vi "Data_get_joe_3.vi"() -> ()   [LabVIEW 2011]
uses:
  <vilib>/Utility/error.llb/DialogType.ctl
  <vilib>/Analysis/2dsp.llb/Real FFT.vi
  <vilib>/Analysis/NI_AALPro.lvlib
panel:
  in  "Automatic Overwrite?":bool
  out "f cur. (GHz)":i32
  in  "TDS VISA Port":refnum<visa-resource-name>="GPIB0::1::INSTR"
  in  "Chirp up to (GHz)":dbl
  in  "PauseB":bool caption="Pause"
  in  "Substr":bool
  out "tdsavges#":i32 caption="tds averaged:"
  in  "Auto":bool caption="Autosave"
  in  "FFT every#":u32=1 min=1 max=1000 step=1
  in  "#steps":u32=1 min=1 step=1
  in  "f step (GHz)":dbl=0.0003 min=0.00025 max=67.0 step=1e-06 format="%#.12f"
  in  "time/point":T1(ring)
  in  "time/div":T2(ring)
  out "Current sweep":u32=1 min=1 max=1000 step=1
  in  "Ext":string="ccd"
  in  "Name":string="trace"
  in  "Folder":path
  in  "#Sweeps":u32=1 min=1 max=1000 step=1
  in  "Ampl. (dBm)":dbl min=-135.0 max=30.0 step=0.5 format="%#_8g"
  in  "f start (GHz)":dbl=0.0003 min=0.00025 max=67.0 step=1e-06 format="%#.12f"
  in  "Start":bool
  in  "Quit":bool
  in  "PSG1 VISA Port":refnum<visa-resource-name>="GPIB0::1::INSTR"
  out "read time (ms)":u32
  out "#points":u32
  out "Busy":bool
  in  "Chirp start (MHz)":ext=2.5
  in  "Filter up to (MHz)":ext=2.5
  in  "Amount of averagings":u32=10 min=1 step=1
  out "Data":dbl[](array[numeric])
  out "Frequency Domain Signal":cluster{ext[], dbl[]}(graph)
  out "FFT (Im)":dbl[](array[numeric])
  out "FFT (Re)":dbl[](array[numeric])
  out "Final array":ext[][](array[numeric])
  out "size(s)":i32
  out "Oscilloscope Data":dbl[](array[numeric])
  in  "Channel Number":u16=1
  out "Oscilloscope graph":dbl[](graph)
  in  "Stop":bool
  # "Oscilloscope TDS6124C"
  # "File Storage"
  # "PSG E8257D"
  # "Control"
  # "Spectrum data"
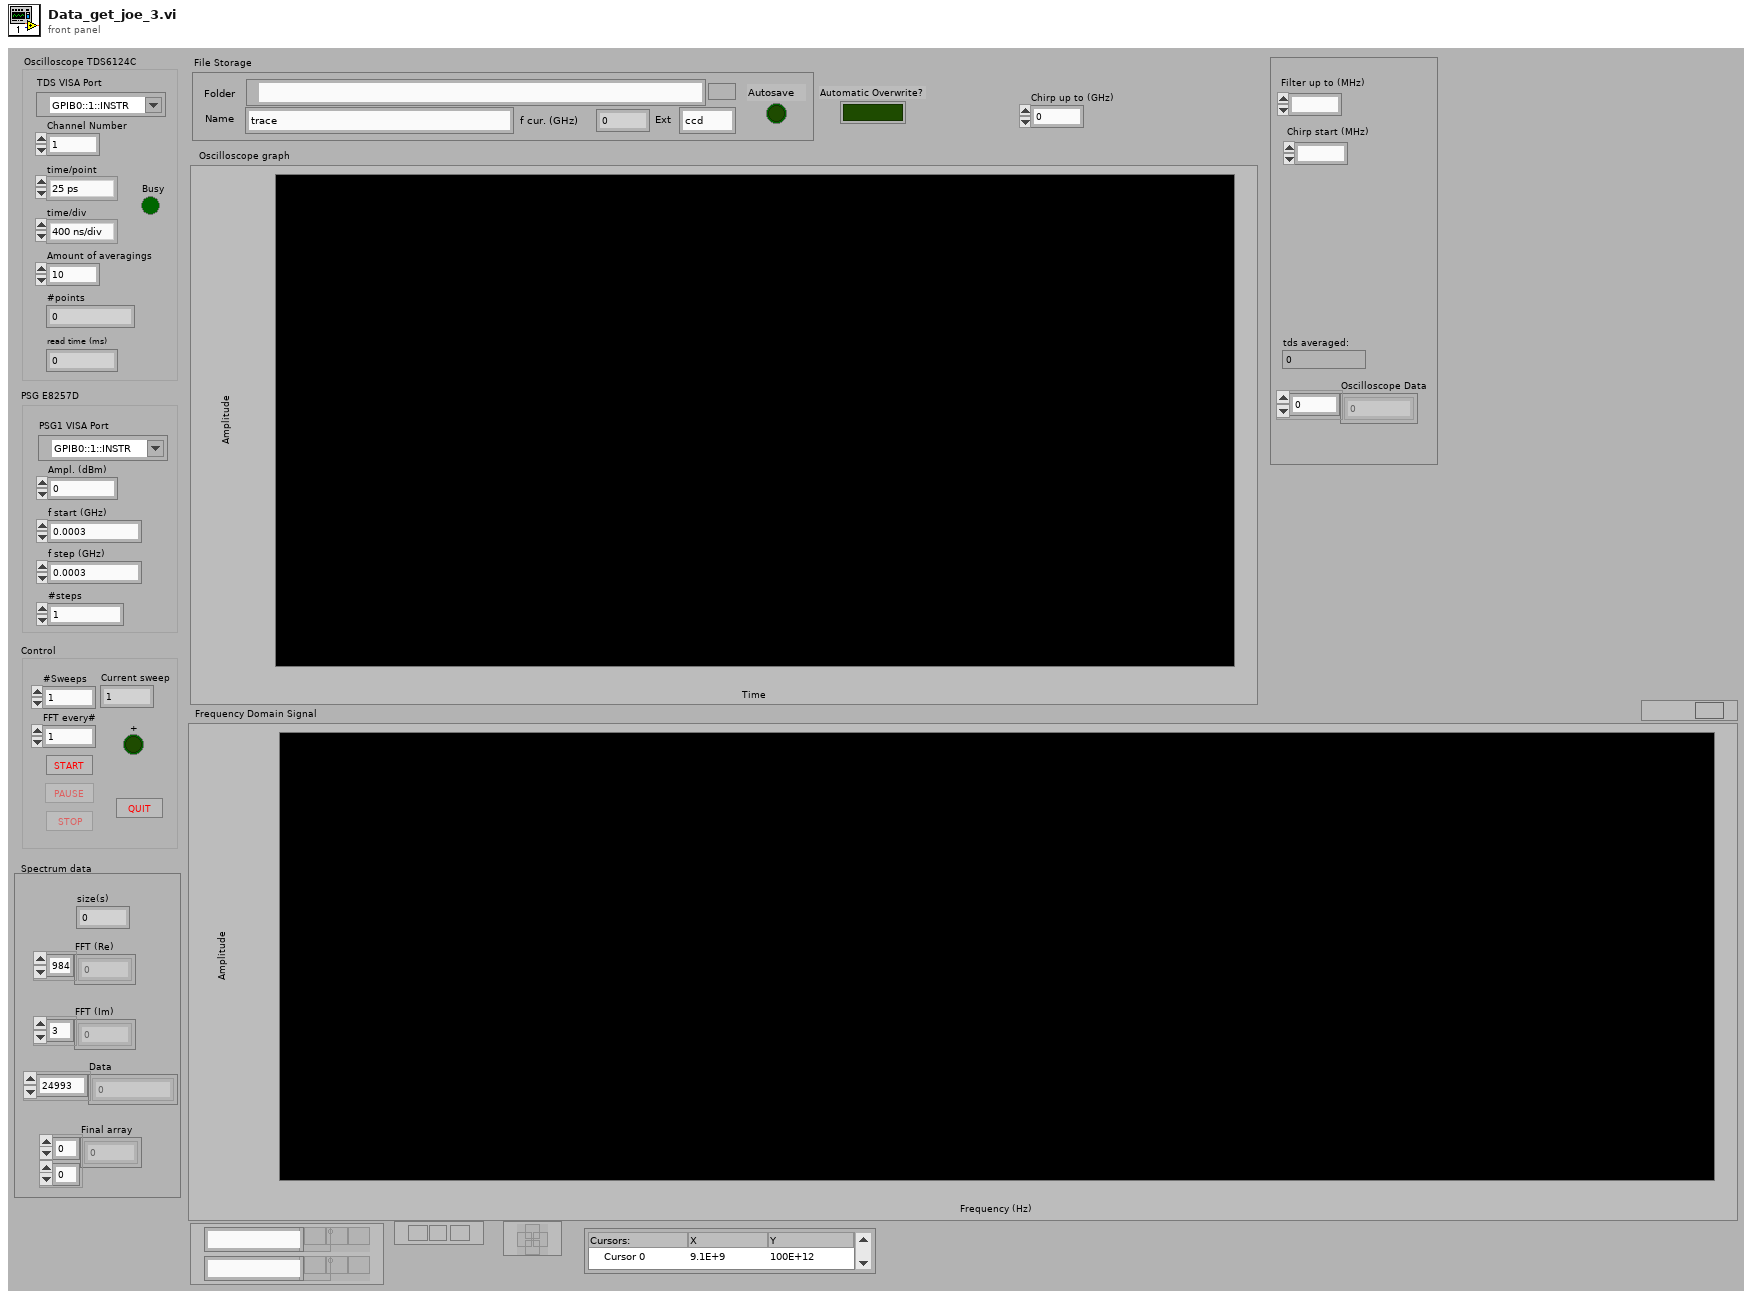
[diagram p1: front panel]
types:
  T1 = enum16{"25 ps", "50 ps", "100 ps", "200 ps", "400 ps", "800 ps", "2 ns"}
  T2 = enum16{"400 ns/div", "1 us/div", "2 us/div", "4 us/div", "10 us/div", "20 us/div"}
  T3 = enum8{"Enabled", "Disabled", "Disabled and Grayed Out"}
  T4 = enum16{"open", "replace", "create", "open or create", "replace or create", "replace or create with confirmation"}
  T5 = typedef "DialogType.ctl" = u16
  T6 = cluster{"Folder":path, "Name":string, "Ext":string}
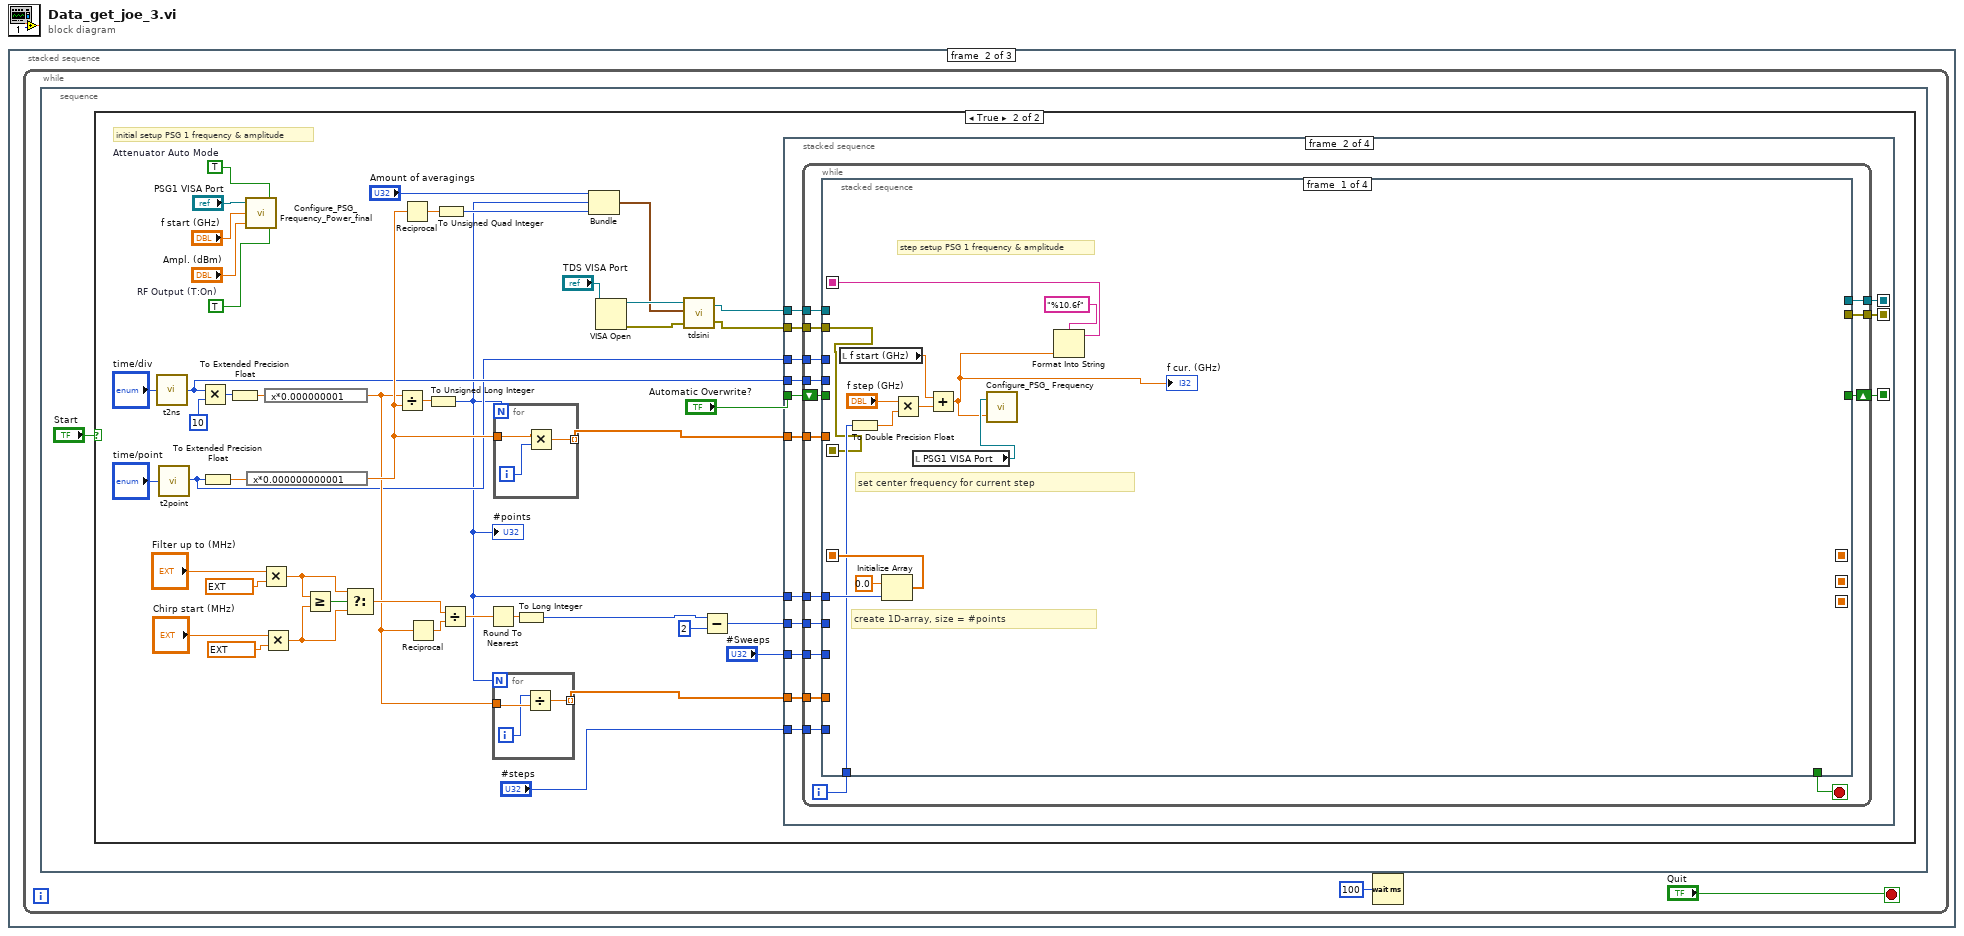
[diagram p0: block diagram]
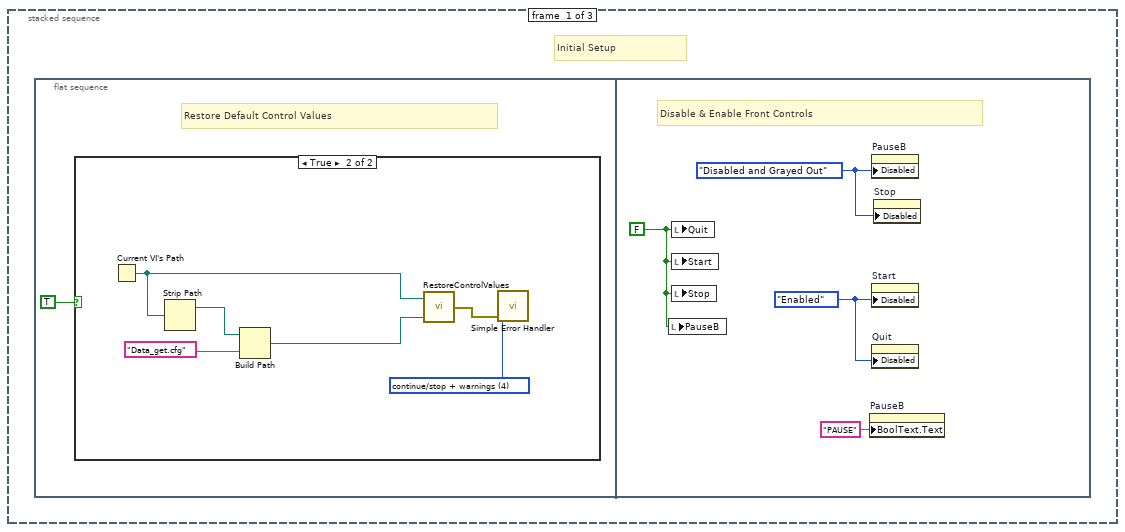
[diagram p2: hidden frame]
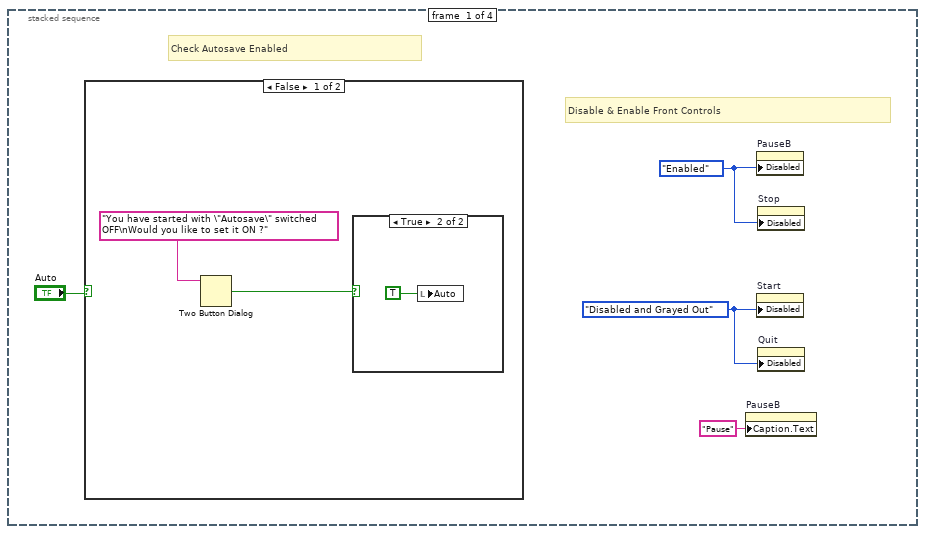
[diagram p5: hidden frame]
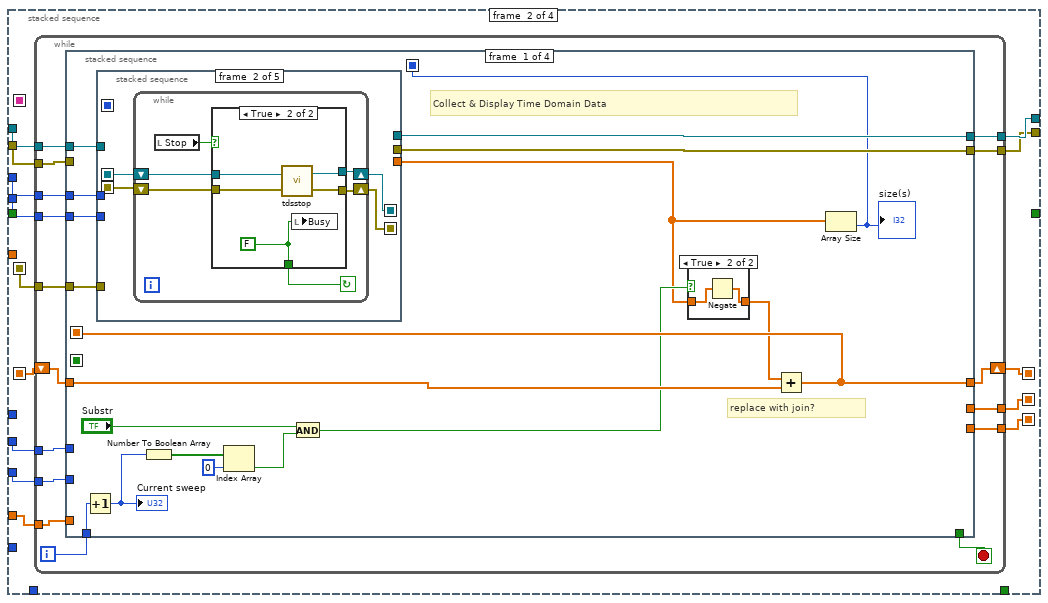
[diagram p8: hidden frame]
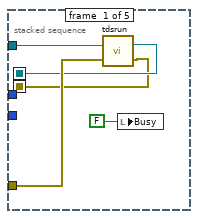
[diagram p10: hidden frame]
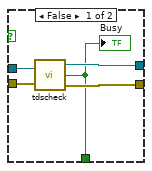
[diagram p11: hidden frame]
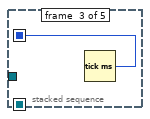
[diagram p12: hidden frame]
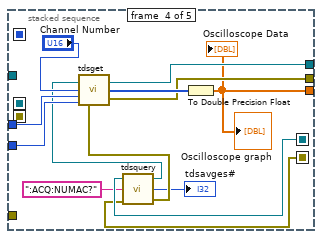
[diagram p13: hidden frame]
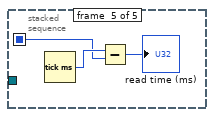
[diagram p14: hidden frame]
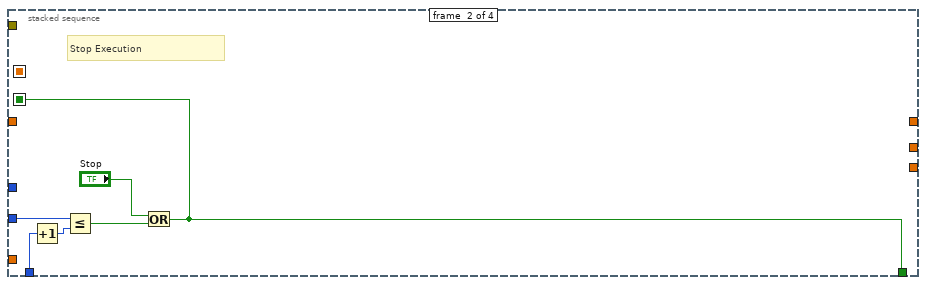
[diagram p15: hidden frame]
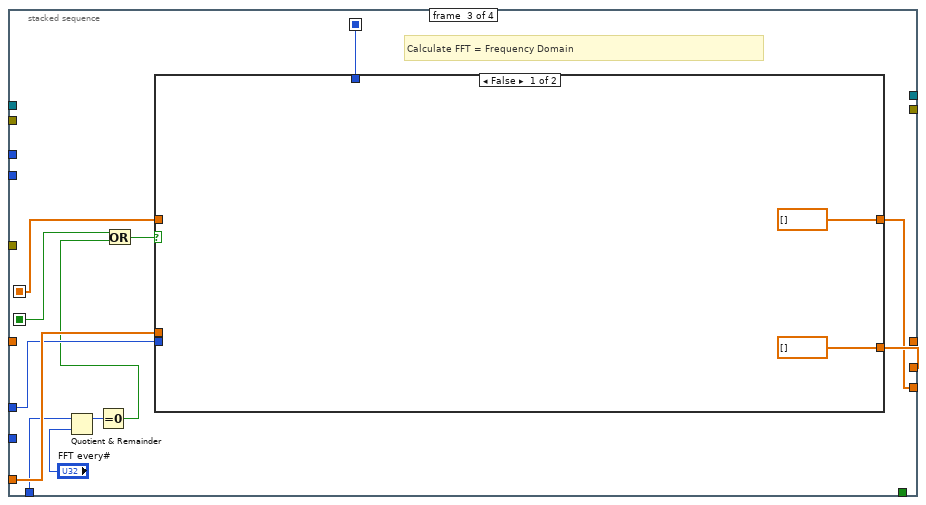
[diagram p16: hidden frame]
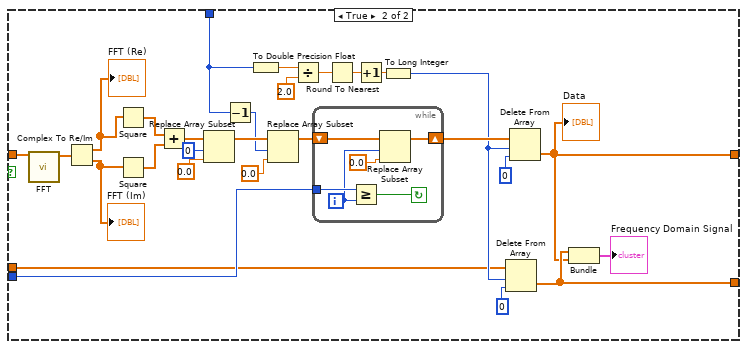
[diagram p17: hidden frame]
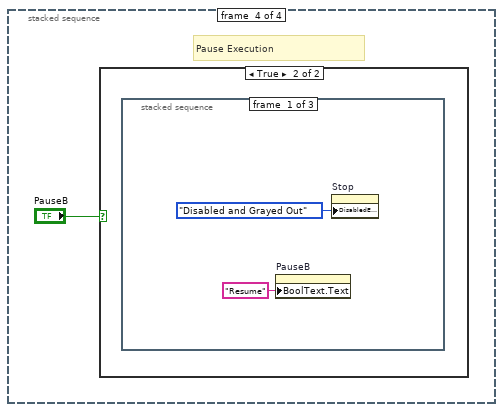
[diagram p18: hidden frame]
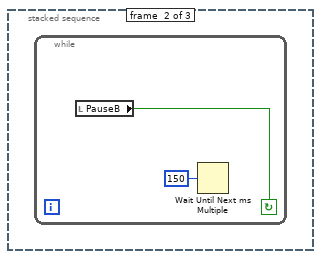
[diagram p20: hidden frame]
diagram:
  n1 = stacked-sequence {
    frame #0 {
      # "Initial Setup"
      n2 = flat-sequence {
        frame #0 {
          # "Restore Default Control Values"
          n3 = case shown="True" TRUE {
            frame False {
            }
            frame True {
              w2 = T5 4 items=["no dialog", "OK message", "continue or stop message", "OK message + warnings", "continue/stop + warnings"] ("type of dialog (OK msg:1)")
              n4 = Current VI's Path() -> (path=w3:path)
              n5 = Strip Path(path=w3) -> (stripped path=w4:path)  [unwired: 1 out]
              n6 = Build Path(base path=w4, name or relative path="Data_get.cfg") -> (appended path=w6:path)
              n7 = call "RestoreControlValues.vi"("file path"=w6, "vi path"=w3) -> ("error out"=w5:errorcluster)
              n8 = call <vilib>:"Simple Error Handler.vi"("type of dialog (OK msg:1)"=w2, "error in (no error)"=w5) -> ()  [unwired: 3 in, 5 out]
            }
          }
        }
        frame #1 {
          w10 = T3."Disabled and Grayed Out" ("Disabled")
          w8 = T3."Enabled" ("Disabled")
          w11 = FALSE ("Quit")
          # "Disable & Enable Front Controls"
          n9 = local write "PauseB"(w11) -> ()
          n10 = local write "Quit"(w11) -> ()
          n11 = local write "Start"(w11) -> ()
          n12 = local write "Stop"(w11) -> ()
          n13 = property on="PauseB" class="Bool (strict)"("BoolText.Text"="PAUSE" ("Boolean Text.Text")) -> ()  [unwired: 2 in, 2 out]
          n14 = property on="PauseB" class="Bool (strict)"("Disabled"=w10) -> ()  [unwired: 2 in, 2 out]
          n15 = property on="Start" class="Bool (strict)"("Disabled"=w8) -> ()  [unwired: 2 in, 2 out]
          n16 = property on="Quit" class="Bool (strict)"("Disabled"=w8) -> ()  [unwired: 2 in, 2 out]
          n17 = property on="Stop" class="Bool (strict)"("Disabled"=w10) -> ()  [unwired: 2 in, 2 out]
        }
      }
    }
    frame #1 {
      n18 = while {
        stop <- "Quit" stop-if-true
        n19 = stacked-sequence {
          frame #0 {
            n20 = case shown="True" "Start" {
              frame False {
              }
              frame True {
                w19 = TRUE  # Attenuator Auto Mode
                w16 = TRUE  # RF Output (T:On)
                # "initial setup PSG 1 frequency & amplitude"
                n21 = call "t2ns.vi"("t/div"="time/div") -> ("ns/div"=w31:u32)
                n22 = call "t2point.vi"("t/point"="time/point") -> ("ps/point"=w29:u32)
                n23 = Multiply(x=w31, y=u32 10) -> (x*y=w54:u32)
                n24 = To Extended Precision Float(1:w29) -> (0:w51:ext)
                n25 = To Extended Precision Float(1:w54) -> (0:w52:ext)
                n26 = call "Configure_PSG_ Frequency_Power_final.vi"("RF Output (T:On)"=w16, "Attenuator Auto Mode (T:Enable)"=w19, "Power [dBm]"="Ampl. (dBm)", "Frequency [GHz]"="f start (GHz)", "VISA resource name"="PSG1 VISA Port") -> ()
                n27 = expression code="x*0.000000000001"(w51) -> (w37:ext)
                n28 = Multiply(x="Filter up to (MHz)", y=ext 1000000.0) -> (x*y=w43:ext)
                n29 = Multiply(x="Chirp start (MHz)", y=ext 1000000.0) -> (x*y=w40:ext)
                n30 = expression code="x*0.000000001"(w52) -> (w33:ext)
                n31 = Greater Or Equal?(x=w43, y=w40) -> (x >= y?=w50:bool)
                n32 = Select(t=w43, s=w50, f=w40) -> (s? t:f=w48:ext)
                n33 = Divide(x=w33, y=w37) -> (x/y=w53:ext)
                n34 = Reciprocal(x=w37) -> (1/x=w35:ext)
                n35 = Reciprocal(x=w33) -> (1/x=w49:ext)
                n36 = To Unsigned Long Integer(number=w53) -> (unsigned 32bit integer=w27:u32)
                "#points" <- w27
                n37 = To Unsigned Quad Integer(1:w35) -> (0:w36:u64)
                n38 = Divide(x=w48, y=w49) -> (x/y=w47:ext)
                n39 = Round To Nearest(number=w47) -> (nearest integer value=w46:ext)
                n40 = for {
                  N: w27 -> [_]
                  tunnel: w33 -> [w455]
                  tunnel: [w456] -> w34 mode=indexing
                  i -> [w454]
                  n41 = Divide(x=w454, y=w455) -> (x/y=w456:ext)
                }
                n42 = for {
                  N: w27 -> [_]
                  tunnel: w37 -> [w459]
                  tunnel: [w458] -> w32 mode=indexing
                  i -> [w457]
                  n43 = Multiply(x=w459, y=w457) -> (x*y=w458:ext)
                }
                n44 = To Long Integer(number=w46) -> (32bit integer=w24:i32)
                n45 = Bundle("Amount of averagings"="Amount of averagings", w27, w36) -> (w38:cluster{"Amount of averagings ":u32, u32, u64})  [unwired: 1 in]
                n46 = VISA Open(VISA resource name="TDS VISA Port") -> (VISA resource name=w56:refnum<visa-resource-name>, error out=w57:errorcluster)  [unwired: 4 in]
                n47 = call "tdsini.vi"("Error In (No Error)"=w57, "Acq_par"=w38, "VISA Port In"=w56) -> ("Error Out"=w58:errorcluster, "VISA Port Out"=w59:refnum<visa-resource-name>)
                n48 = Subtract(x=w24, y=2) -> (x-y=w22:i32)
                n49 = stacked-sequence {
                  seq-local: [_ w73 _ _] -> [_ _ w415 _]
                  seq-local: [_ w72 _ _] -> [_ _ w414 _]
                  seq-local: [_ w67 _ _] -> [_ _ _ w416]
                  tunnel: w59 -> [_ w80 _ _]
                  tunnel: w58 -> [_ w79 _ _]
                  tunnel: w29 -> [_ w78 _ _]
                  tunnel: w31 -> [_ w77 _ _]
                  tunnel: w22 -> [_ w76 _ _]
                  tunnel: w34 -> [_ w75 _ _]
                  tunnel: "#Sweeps" -> [_ w74 _ _]
                  tunnel: w32 -> [_ w69 _ _]
                  tunnel: w27 -> [_ w71 _ _]
                  tunnel: "#steps" -> [_ w70 _ _]
                  tunnel: "Automatic Overwrite?" -> [_ w68 _ _]
                  frame #0 {
                    w61 = T3."Enabled" ("Disabled")
                    w60 = T3."Disabled and Grayed Out" ("Disabled")
                    # "Check Autosave Enabled"
                    # "Disable & Enable Front Controls"
                    n50 = case shown="False" "Auto" {
                      frame False {
                        n51 = Two Button Dialog(message="You have started with \"Autosave\" switched OFF\nWould you like to set it ON ?") -> (T button?=w64:bool)  [unwired: 2 in]
                        n52 = case shown="True" w64 {
                          frame False {
                          }
                          frame True {
                            n53 = local write "Auto"(TRUE) -> ()
                          }
                        }
                      }
                      frame True {
                      }
                    }
                    n54 = property on="PauseB" class="Bool (strict)"("Caption.Text"="Pause") -> ()  [unwired: 2 in, 2 out]
                    n55 = property on="PauseB" class="Bool (strict)"("Disabled"=w61) -> ()  [unwired: 2 in, 2 out]
                    n56 = property on="Start" class="Bool (strict)"("Disabled"=w60) -> ()  [unwired: 2 in, 2 out]
                    n57 = property on="Stop" class="Bool (strict)"("Disabled"=w61) -> ()  [unwired: 2 in, 2 out]
                    n58 = property on="Quit" class="Bool (strict)"("Disabled"=w60) -> ()  [unwired: 2 in, 2 out]
                  }
                  frame #1 {
                    n59 = while {
                      tunnel: w80 -> [w96]
                      tunnel: w79 -> [w95]
                      tunnel: w78 -> [w94]
                      tunnel: w77 -> [w93]
                      tunnel: w76 -> [w92]
                      tunnel: w75 -> [w91]
                      tunnel: w74 -> [w90]
                      tunnel: [w89] -> w73
                      tunnel: [w88] -> w72
                      tunnel: w71 -> [w87]
                      tunnel: w70 -> [w85]
                      tunnel: w69 -> [w83]
                      shift-right: [w81] -> w67
                      shift-left: w68 -> [w82]
                      i -> [w86]
                      stop <- w84 stop-if-true
                      n60 = stacked-sequence {
                        seq-local: [w108 _ _ _] -> [_ w114 _ _]
                        seq-local: [w99 _ _ _] -> [_ w113 _ _]
                        seq-local: [_ w112 _ _] -> [_ _ w270 _]
                        seq-local: [_ w111 _ _] -> [_ _ w269 _]
                        seq-local: [_ w110 _ _] -> [_ _ w268 _]
                        seq-local: [w100 _ _ _] -> [_ _ w267 _]
                        tunnel: w96 -> [_ w123 _ _]
                        tunnel: w95 -> [w99 w122 _ _]
                        tunnel: w94 -> [_ w121 _ _]
                        tunnel: w93 -> [_ w120 _ _]
                        tunnel: w92 -> [_ w119 _ _]
                        tunnel: w91 -> [_ w118 _ _]
                        tunnel: w90 -> [_ w117 _ _]
                        tunnel: [_ w116 _ _] -> w89
                        tunnel: [_ w115 _ _] -> w88
                        tunnel: w87 -> [w107 _ _ _]
                        tunnel: w86 -> [w104 _ _ w408]
                        tunnel: w85 -> [_ _ _ w407]
                        tunnel: [_ _ _ w406] -> w84
                        tunnel: w83 -> [_ _ w271 _]
                        tunnel: w82 -> [_ _ w265 _]
                        tunnel: [_ _ w264 _] -> w81
                        frame #0 {
                          # "step setup PSG 1 frequency & amplitude"
                          # "create 1D-array, size = #points"
                          # "set center frequency for current step"
                          n61 = local read "f start (GHz)"() -> (w102:dbl)
                          n62 = To Double Precision Float(number=w104) -> (double precision float=w105:dbl)
                          n63 = Initialize Array(0.0 ("element"), w107) -> (w108:dbl[])
                          n64 = Multiply(x="f step (GHz)", y=w105) -> (x*y=w103:dbl)
                          n65 = local read "PSG1 VISA Port"() -> (w98:refnum<visa-resource-name>)
                          n66 = Add(x=w102, y=w103) -> (x+y=w97:dbl)
                          "f cur. (GHz)" <- w97
                          n67 = call "Configure_PSG_ Frequency.vi"("Frequency [GHz]"=w97, "VISA resource name"=w98) -> ()  [unwired: 1 in]
                          n68 = Format Into String(format string="%10.6f", w97) -> (resulting string=w100:string)  [unwired: 2 in, 1 out]
                        }
                        frame #1 {
                          n69 = while {
                            tunnel: [w136] -> w115
                            tunnel: [w137] -> w116
                            tunnel: w122 -> [w138]
                            tunnel: w123 -> [w139]
                            tunnel: w121 -> [w135]
                            tunnel: w120 -> [w134]
                            tunnel: w118 -> [w132]
                            tunnel: w119 -> [w133]
                            tunnel: w117 -> [w129]
                            shift-right: [w127] -> w112
                            shift-left: w114 -> [w128]
                            tunnel: [w126] -> w111
                            tunnel: w113 -> [w125]
                            tunnel: [w124] -> w110
                            i -> [w131]
                            stop <- w130 stop-if-true
                            n70 = stacked-sequence {
                              seq-local: [w149 _ _ _] -> [_ _ w220 _]
                              seq-local: [w150 _ _ _] -> [_ _ w219 _]
                              seq-local: [_ w203 _ _] -> [_ _ w210 _]
                              tunnel: w139 -> [w157 _ _ _]
                              tunnel: w138 -> [_ _ _ _]
                              tunnel: [w156 _ _ _] -> w137
                              tunnel: [w155 _ _ _] -> w136
                              tunnel: w135 -> [w154 _ _ _]
                              tunnel: w134 -> [w153 _ _ _]
                              tunnel: w133 -> [_ _ w217 _]
                              tunnel: w132 -> [_ _ w218 _]
                              tunnel: w131 -> [w148 w208 w214 _]
                              tunnel: [_ w203 _ _] -> w130
                              tunnel: w129 -> [_ w205 _ _]
                              tunnel: w128 -> [w152 _ _ _]
                              tunnel: [w150 _ _ _] -> w127
                              tunnel: [_ _ w216 _] -> w126
                              tunnel: w125 -> [w151 _ _ _]
                              tunnel: [_ _ w215 _] -> w124
                              frame #0 {
                                # "replace with join?"
                                # "Collect & Display Time Domain Data"
                                n71 = Increment(x=w148) -> (x+1=w140:i32)
                                "Current sweep" <- w140
                                n72 = stacked-sequence {
                                seq-local: [w163 _ _ _ _] -> [_ w169 _ _ _]
                                seq-local: [w162 _ _ _ _] -> [_ w168 _ _ _]
                                seq-local: [_ w166 _ _ _] -> [_ _ _ w191 _]
                                seq-local: [_ w167 _ _ _] -> [_ _ _ w192 _]
                                seq-local: [_ _ w186 _ _] -> [_ _ _ _ w201]
                                tunnel: w157 -> [w164 _ _ _ _]
                                tunnel: w151 -> [w165 _ _ _ _]
                                tunnel: [_ _ _ w198 _] -> w156
                                tunnel: [_ _ _ w197 _] -> w155
                                tunnel: w154 -> [_ _ _ w195 _]
                                tunnel: w153 -> [_ _ _ w194 _]
                                tunnel: [_ _ _ w193 _] -> w143
                                frame #0 {
                                n73 = call "tdsrun.vi"("Error In (No Error)"=w165, "VISA Port In"=w164) -> ("Error Out"=w162:errorcluster, "VISA Port Out"=w163:refnum<visa-resource-name>)
                                n74 = local write "Busy"(FALSE ("Busy")) -> ()
                                }
                                frame #1 {
                                n75 = while {
                                shift-right: [w173] -> w167
                                shift-left: w169 -> [w174]
                                shift-right: [w172] -> w166
                                shift-left: w168 -> [w175]
                                stop <- w171 continue-if-true
                                n76 = local read "Stop"() -> (w170:bool)
                                n77 = case shown="True" w170 {
                                tunnel: w175 -> [w180 w184]
                                tunnel: w174 -> [w179 w185]
                                tunnel: [w178 w182] -> w173
                                tunnel: [w177 w183] -> w172
                                tunnel: [w176 w181] -> w171
                                frame False {
                                n78 = call "tdscheck.vi"("VISA Port In"=w179, "Error In (No Error)"=w180) -> ("VISA Port Out"=w178:refnum<visa-resource-name>, "busy"=w176:bool, "Error Out"=w177:errorcluster)
                                "Busy" <- w176
                                }
                                frame True {
                                w181 = FALSE ("busy")
                                n79 = call "tdsstop.vi"("Error In (No Error)"=w184, "VISA Port In"=w185) -> ("Error Out"=w183:errorcluster, "VISA Port Out"=w182:refnum<visa-resource-name>)
                                n80 = local write "Busy"(w181) -> ()
                                }
                                }
                                }
                                }
                                frame #2 {
                                n81 = Tick Count (ms)() -> (millisecond timer value=w186:u32)
                                }
                                frame #3 {
                                n82 = call "tdsquery.vi"("Error In (No Error)"=w191, "String to TDS"=":ACQ:NUMAC?", "VISA Port In"=w192) -> ("Error Out"=w188:errorcluster, "number"=→"tdsavges#":i32, "VISA Port Out"=w189:refnum<visa-resource-name>)
                                n83 = call "tdsget.vi"("VISA Port In"=w189, "Channel Number"="Channel Number", "ps/point"=w195, "ns/div"=w194, "Error In (No Error)"=w188) -> ("VISA Port Out"=w198:refnum<visa-resource-name>, "TDS Data"=w199:u16[], "Error Out"=w197:errorcluster)  [unwired: 8 in]
                                n84 = To Double Precision Float(number=w199) -> (double precision float=w193:dbl[])
                                "Oscilloscope graph" <- w193
                                "Oscilloscope Data" <- w193
                                }
                                frame #4 {
                                n85 = Tick Count (ms)() -> (millisecond timer value=w202:u32)
                                n86 = Subtract(x=w202, y=w201) -> (x-y=→"read time (ms)":u32)
                                }
                                }
                                n87 = Number To Boolean Array(number=w140) -> (Boolean array=w147:bool[])
                                n88 = Index Array(array=w147, index=0) -> (element=w145:bool)
                                n89 = And(x="Substr", y=w145) -> (x .and. y?=w144:bool)
                                n90 = case shown="True" w144 {
                                tunnel: w143 -> [w158 w160]
                                tunnel: [w158 w159] -> w142
                                frame False {
                                }
                                frame True {
                                n91 = Negate(x=w160) -> (-x=w159:dbl[])
                                }
                                }
                                n92 = Add(x=w142, y=w152) -> (x+y=w150:dbl[])
                                n93 = Array Size(array=w143) -> (size(s)=w149:i32)
                                "size(s)" <- w149
                              }
                              frame #1 {
                                # "Stop Execution"
                                n94 = Increment(x=w208) -> (x+1=w204:i32)
                                n95 = Less Or Equal?(x=w205, y=w204) -> (x <= y?=w207:bool)
                                n96 = Or(x="Stop", y=w207) -> (x .or. y?=w203:bool)
                              }
                              frame #2 {
                                # "Calculate FFT = Frequency Domain"
                                n97 = Quotient & Remainder(x=w214, y="FFT every#") -> (x-y*floor(x/y)=w212:u32)  [unwired: 1 out]
                                n98 = Equal To 0?(x=w212) -> (x = 0?=w209:bool)
                                n99 = Or(x=w210, y=w209) -> (x .or. y?=w211:bool)
                                n100 = case shown="False" w211 {
                                tunnel: w220 -> [_ w228]
                                tunnel: w219 -> [_ w227]
                                tunnel: w218 -> [_ w223]
                                tunnel: w217 -> [_ w226]
                                tunnel: [ext[] [] w225] -> w216
                                tunnel: [dbl[] [] w224] -> w215
                                frame False {
                                }
                                frame True {
                                n101 = call-poly <vilib>:"FFT.vi"("X"=w227) -> ("FFT {X}"=w250:cdb[])  [unwired: 9 in, 1 out]
                                n102 = Complex To Re/Im(x + iy=w250) -> (x=w249:dbl[], y=w248:dbl[])
                                "FFT (Re)" <- w249
                                "FFT (Im)" <- w248
                                n103 = Square(x=w249) -> (x^2=w247:dbl[])
                                n104 = Square(x=w248) -> (x^2=w246:dbl[])
                                n105 = Add(x=w247, y=w246) -> (x+y=w242:dbl[])
                                n106 = Replace Array Subset(array=w242, new element=0.0 ("new element/subarray"), index=0) -> (w241:dbl[])
                                n107 = Decrement(x=w228) -> (x-1=w240:i32)
                                n108 = To Double Precision Float(number=w228) -> (double precision float=w236:dbl)
                                n109 = Replace Array Subset(array=w241, new element=0.0 ("new element/subarray"), index=w240) -> (w238:dbl[])
                                n110 = Divide(x=w236, y=2.0) -> (x/y=w234:dbl)
                                n111 = while {
                                tunnel: w226 -> [w255]
                                shift-right: [w253] -> w237
                                shift-left: w238 -> [w254]
                                i -> [w252]
                                stop <- w256 continue-if-true
                                n112 = Greater Or Equal?(x=w255, y=w252) -> (x >= y?=w256:bool)
                                n113 = Replace Array Subset(array=w254, new element=0.0 ("new element/subarray"), index=w252) -> (w253:dbl[])
                                }
                                n114 = Round To Nearest(number=w234) -> (nearest integer value=w233:dbl)
                                n115 = Increment(x=w233) -> (x+1=w232:dbl)
                                n116 = To Long Integer(number=w232) -> (32bit integer=w229:i32)
                                n117 = Delete From Array(array=w223, length=w229, index=0) -> (deleted portion=w225:ext[])  [unwired: 1 out]
                                n118 = Delete From Array(array=w237, length=w229, index=0) -> (deleted portion=w224:dbl[])  [unwired: 1 out]
                                "Data" <- w224
                                n119 = Bundle(w225, w224) -> (→"Frequency Domain Signal":cluster{ext[], dbl[]})  [unwired: 1 in]
                                }
                                }
                              }
                              frame #3 {
                                # "Pause Execution"
                                n120 = case shown="True" "PauseB" {
                                frame False {
                                }
                                frame True {
                                n121 = stacked-sequence {
                                frame #0 {
                                n122 = property on="PauseB" class="Bool (strict)"("BoolText.Text"="Resume" ("Caption.Text")) -> ()  [unwired: 2 in, 2 out]
                                n123 = property on="Stop" class="Bool (strict)"("DisabledEnum"=T3."Disabled and Grayed Out" ("Disabled")) -> ()  [unwired: 2 in, 2 out]
                                }
                                frame #1 {
                                n124 = while {
                                stop <- w261 continue-if-true
                                n125 = local read "PauseB"() -> (w261:bool)
                                n126 = Wait Until Next ms Multiple(millisecond multiple=u32 150) -> ()  [unwired: 1 out]
                                }
                                }
                                frame #2 {
                                n127 = property on="PauseB" class="Bool (strict)"("BoolText.Text"="Pause" ("Caption.Text")) -> ()  [unwired: 2 in, 2 out]
                                n128 = property on="Stop" class="Bool (strict)"("DisabledEnum"=T3."Enabled" ("Disabled")) -> ()  [unwired: 2 in, 2 out]
                                }
                                }
                                }
                                }
                              }
                            }
                          }
                        }
                        frame #2 {
                          # "Auto Safe?"
                          n129 = local read "Auto"() -> (w266:bool)
                          n130 = case shown="True" w266 {
                            tunnel: w271 -> [_ w279]
                            tunnel: w270 -> [_ w278]
                            tunnel: w269 -> [_ w277]
                            tunnel: w268 -> [_ w276]
                            tunnel: w267 -> [_ w275]
                            tunnel: w265 -> [_ w274]
                            tunnel: [FALSE w273] -> w264
                            frame False {
                            }
                            frame True {
                              n131 = stacked-sequence {
                                seq-local: [w280 _ _ _] -> [_ w304 _ _]
                                seq-local: [_ _ w358 _] -> [_ _ _ w398]
                                seq-local: [_ w290 _ _] -> [_ _ _ w389]
                                tunnel: w279 -> [_ w306 _ _]
                                tunnel: w278 -> [_ w293 _ _]
                                tunnel: w277 -> [_ _ _ w401]
                                tunnel: w276 -> [_ _ _ w400]
                                tunnel: w275 -> [w283 w292 w360 _]
                                tunnel: w274 -> [_ w296 _ _]
                                tunnel: [_ w290 _ _] -> w273
                                frame #0 {
                                # "create complete filename incl. path as a string"
                                n132 = Path To String(path="Folder") -> (string=w288:string)
                                n133 = Concatenate Strings(w288, "\\\\" ("string"), "Name", "_", "td", w283, ".", "Ext") -> (w280:string)
                                }
                                frame #1 {
                                # "(%e) = Scientific Notation"
                                n134 = Build Array(w306, w293) -> (w308:ext[][])
                                n135 = String To Path(string=w304) -> (path=w295:path)
                                n136 = case shown="False" w296 {
                                tunnel: w304 -> [w310 _]
                                tunnel: [w315 w356] -> w290
                                tunnel: [w313 T4."replace or create" ("operation (0:open)")] -> w298
                                tunnel: w296 -> [w314 w356]
                                tunnel: w295 -> [w312 w355]
                                tunnel: [w311 w355] -> w294
                                tunnel: w292 -> [w309 _]
                                frame False {
                                n137 = call "CheckFileExist.vi"("Path"=w310) -> ("File Exists"=w317:bool, "Overwrite File"=w316:bool)  [unwired: 1 in, 1 out]
                                n138 = case "check file existance" shown="True" w317 {
                                tunnel: w316 -> [_ w326]
                                tunnel: [w320 w324] -> w315
                                tunnel: w314 -> [w320 _]
                                tunnel: [T4."create" ("operation (0:open)") w325] -> w313
                                tunnel: w312 -> [w318 w323]
                                tunnel: [w318 w322] -> w311
                                tunnel: w309 -> [_ w321]
                                frame False {
                                # "file doesn't exist"
                                }
                                frame True {
                                # "file exists"
                                n139 = case shown="False" w326 {
                                tunnel: [w329 T4."replace or create" ("operation (0:open)")] -> w325
                                tunnel: [w330 TRUE] -> w324
                                tunnel: w323 -> [_ w352]
                                tunnel: [w327 w352] -> w322
                                tunnel: w321 -> [w328 _]
                                frame False {
                                # "file exists and should not be overwritten"
                                n140 = stacked-sequence {
                                tunnel: [_ _ FALSE] -> w330
                                tunnel: [_ _ T4."create" ("operation (0:open)")] -> w329
                                tunnel: w328 -> [_ w339 _]
                                tunnel: [_ w344 _] -> w327
                                frame #0 {
                                # "enter new file name"
                                n141 = local read "Folder"() -> (w338:path)
                                n142 = local read "Name"() -> (w337:string)
                                n143 = local read "Ext"() -> (w336:string)
                                n144 = Bundle("Folder"=w338, "Name"=w337, "Ext"=w336) -> (w335:T6)  [unwired: 1 in]
                                n145 = call "ChangeFileName.vi"("input par"=w335) -> ("output par"=w334:T6)  [unwired: 1 out]
                                n146 = Unbundle(w334) -> ("Folder"=w333:path, "Name"=w332:string, "Ext"=w331:string)
                                n147 = local write "Folder"(w333) -> ()
                                n148 = local write "Name"(w332) -> ()
                                n149 = local write "Ext"(w331) -> ()
                                }
                                frame #1 {
                                # "create new path"
                                n150 = local read "Ext"() -> (w341:string)
                                n151 = local read "Folder"() -> (w346:path)
                                n152 = local read "Name"() -> (w345:string)
                                n153 = Path To String(path=w346) -> (string=w349:string)
                                n154 = Concatenate Strings(w349, "\\\\" ("string"), w345, "_", "td", w339, ".", w341) -> (w340:string)
                                n155 = String To Path(string=w340) -> (path=w344:path)
                                }
                                frame #2 {
                                }
                                }
                                }
                                frame True {
                                # "overwrite existing file"
                                }
                                }
                                }
                                }
                                }
                                frame True {
                                }
                                }
                                n156 = Transpose 2D Array(2D array=w308) -> (transposed array=w305:ext[][])
                                n157 = Array To Spreadsheet String(array=w305, 3:"%e") -> (spreadsheet string=w297:string)  [unwired: 1 in]
                                n158 = Open/Create/Replace File(file path (use dialog)=w294, operation (0:open)=w298, access (0:read/write)=enum16{"read/write", "read-only", "write-only"}."write-only") -> (refnum out=w300:refnum<file>, error out=w303:errorcluster)  [unwired: 3 in, 1 out]
                                n159 = Write to Text File(file (use dialog)=w300, text=w297, error in=w303) -> (refnum out=w301:refnum<file>, error out=w302:errorcluster)  [unwired: 1 in, 1 out]
                                n160 = Close File(refnum=w301, error in=w302) -> (error out=w291:errorcluster)  [unwired: 1 out]
                                n161 = call <vilib>:"Simple Error Handler.vi"("error in (no error)"=w291) -> ()  [unwired: 4 in, 5 out]
                                }
                                frame #2 {
                                n162 = local read "Folder"() -> (w362:path)
                                n163 = local read "Name"() -> (w361:string)
                                n164 = local read "Ext"() -> (w359:string)
                                n165 = Path To String(path=w362) -> (string=w368:string)
                                n166 = Concatenate Strings(w368, "\\\\" ("string"), w361, "_") -> (w363:string)
                                n167 = Concatenate Strings(w363, "sd", w360, ".", w359) -> (w358:string)
                                }
                                frame #3 {
                                n168 = Multiply(x="Chirp up to (GHz)", y=1000000000.0) -> (x*y=w370:dbl)
                                n169 = To Extended Precision Float(1:w370) -> (0:w369:ext)
                                n170 = To Extended Precision Float(1:w400) -> (0:w402:ext[])
                                n171 = Build Array(w401, w402) -> (w399:ext[][])
                                n172 = String To Path(string=w398) -> (path=w391:path)
                                n173 = case shown="True" w389 {
                                tunnel: [T4."replace or create with confirmation" ("operation (0:open)") T4."replace or create" ("operation (0:open)")] -> w390
                                frame False {
                                }
                                frame True {
                                }
                                }
                                n174 = Transpose 2D Array(2D array=w399) -> (transposed array=w372:ext[][])
                                n175 = Index Array(array=w372, index (col)=0 ("disabled index (col)")) -> (element=w382:ext[])  [unwired: 1 in]
                                n176 = Index Array(array=w382, index=1) -> (element=w384:ext)
                                n177 = Index Array(array=w382, index=0) -> (element=w383:ext)
                                n178 = Subtract(x=w384, y=w383) -> (x-y=w379:ext)
                                n179 = Divide(x=w369, y=w379) -> (x/y=w376:ext)
                                n180 = Round To Nearest(number=w376) -> (nearest integer value=w378:ext)
                                n181 = To Long Integer(number=w378) -> (32bit integer=w377:i32)
                                n182 = Increment(x=w377) -> (x+1=w373:i32)
                                n183 = Array Subset(array=w372, index (row)=0 ("index"), length (row)=w373, index (col)=0 ("index"), length (col)=w373) -> (w371:ext[][])
                                "Final array" <- w371
                                n184 = Array To Spreadsheet String(array=w371, 3:"%e") -> (spreadsheet string=w392:string)  [unwired: 1 in]
                                n185 = Open/Create/Replace File(file path (use dialog)=w391, operation (0:open)=w390, access (0:read/write)=enum16{"read/write", "read-only", "write-only"}."write-only") -> (refnum out=w394:refnum<file>, error out=w397:errorcluster)  [unwired: 3 in, 1 out]
                                n186 = Write to Text File(file (use dialog)=w394, text=w392, error in=w397) -> (refnum out=w395:refnum<file>, error out=w396:errorcluster)  [unwired: 1 in, 1 out]
                                n187 = Close File(refnum=w395, error in=w396) -> (error out=w388:errorcluster)  [unwired: 1 out]
                                n188 = call <vilib>:"Simple Error Handler.vi"("error in (no error)"=w388) -> ()  [unwired: 4 in, 5 out]
                                }
                              }
                            }
                          }
                        }
                        frame #3 {
                          n189 = Increment(x=w408) -> (x+1=w410:i32)
                          n190 = Less Or Equal?(x=w407, y=w410) -> (x <= y?=w411:bool)
                          n191 = local read "Stop"() -> (w409:bool)
                          n192 = Or(x=w409, y=w411) -> (x .or. y?=w406:bool)
                        }
                      }
                    }
                  }
                  frame #2 {
                    w413 = T3."Disabled and Grayed Out" ("Disabled")
                    w412 = T3."Enabled" ("Disabled")
                    n193 = property on="Quit" class="Bool (strict)"("Disabled"=w412) -> ()  [unwired: 2 in, 2 out]
                    n194 = property on="PauseB" class="Bool (strict)"("Disabled"=w413) -> ()  [unwired: 2 in, 2 out]
                    n195 = property on="Stop" class="Bool (strict)"("Disabled"=w413) -> ()  [unwired: 2 in, 2 out]
                    n196 = property on="Start" class="Bool (strict)"("Disabled"=w412) -> ()  [unwired: 2 in, 2 out]
                    n197 = VISA Close(VISA resource name=w415, error in (no error)=w414) -> ()  [unwired: 1 out]
                  }
                  frame #3 {
                    n198 = local read "Auto"() -> (w417:bool)
                    n199 = case shown="True" w417 {
                      tunnel: w416 -> [_ w420]
                      frame False {
                      }
                      frame True {
                        # "safe measurement settings to file"
                        n200 = local read "time/point"() -> (w449:T1)
                        n201 = local read "time/div"() -> (w448:T2)
                        n202 = local read "Channel Number"() -> (w450:u16)
                        n203 = local read "Amount of averagings"() -> (w447:u32)
                        n204 = local read "#Sweeps"() -> (w446:u32)
                        n205 = local read "Filter up to (MHz)"() -> (w445:ext)
                        n206 = local read "Chirp start (MHz)"() -> (w444:ext)
                        n207 = local read "Ampl. (dBm)"() -> (w443:dbl)
                        n208 = local read "f start (GHz)"() -> (w440:dbl)
                        n209 = local read "f step (GHz)"() -> (w439:dbl)
                        n210 = local read "#steps"() -> (w438:u32)
                        n211 = call "t2point.vi"("t/point"=w449) -> ("ps/point"=w441:u32)
                        n212 = call "t2ns.vi"("t/div"=w448) -> ("ns/div"=w442:u32)
                        n213 = local read "Folder"() -> (w434:path)
                        n214 = local read "Name"() -> (w433:string)
                        n215 = local read "Ext"() -> (w430:string)
                        n216 = Path To String(path=w434) -> (string=w437:string)
                        n217 = Format Into String(format string="Channel: %d\\nps/point: %d\\nns/div: %d\\nAmount of averagings: %d\\n#Sweeps: %d\\nFilter up to (MHz): %f\\nChirp start (MHz): %f\\nAmpl. (dBm): %f\\nf start (GHz): %f\\nf step (MHz): %f\\n#steps: %d\\n", w450, w441, w442, w447, w446, w445, w444, w443, w440, w439, w438) -> (resulting string=w421:string)  [unwired: 2 in, 1 out]
                        n218 = case shown="True" w420 {
                          tunnel: [T4."replace or create with confirmation" ("operation (0:open)") T4."replace or create" ("operation (0:open)")] -> w419
                          frame False {
                          }
                          frame True {
                          }
                        }
                        n219 = Concatenate Strings(w437, "\\\\" ("string"), w433, "_", "par", ".", w430) -> (w429:string)
                        n220 = String To Path(string=w429) -> (path=w423:path)
                        n221 = Open/Create/Replace File(file path (use dialog)=w423, operation (0:open)=w419, access (0:read/write)=enum16{"read/write", "read-only", "write-only"}."write-only") -> (refnum out=w425:refnum<file>, error out=w428:errorcluster)  [unwired: 3 in, 1 out]
                        n222 = Write to Text File(file (use dialog)=w425, text=w421, error in=w428) -> (refnum out=w426:refnum<file>, error out=w427:errorcluster)  [unwired: 1 in, 1 out]
                        n223 = Close File(refnum=w426, error in=w427) -> (error out=w424:errorcluster)  [unwired: 1 out]
                        n224 = call <vilib>:"Simple Error Handler.vi"("error in (no error)"=w424) -> ()  [unwired: 4 in, 5 out]
                      }
                    }
                    n225 = local write "Stop"(FALSE ("Stop")) -> ()
                  }
                }
              }
            }
          }
        }
        n226 = Wait (ms)(milliseconds to wait=u32 100) -> ()  [unwired: 1 out]
      }
    }
    frame #2 {
      n227 = Current VI's Path() -> (path=w460:path)
      n228 = Strip Path(path=w460) -> (stripped path=w461:path)  [unwired: 1 out]
      n229 = Build Path(base path=w461, name or relative path="Data_get.cfg") -> (appended path=w463:path)
      n230 = call "SaveControlValues.vi"("file path"=w463, "vi path"=w460) -> ("error out"=w462:errorcluster)
      n231 = call <vilib>:"Simple Error Handler.vi"("error in (no error)"=w462) -> ()  [unwired: 4 in, 5 out]
    }
  }
